vi "create subregions.vi"(8 "error in (no error)":errorcluster, 11 "Autofocus in":refnum<class "Autofocus.lvclass">) -> (0 "error out":errorcluster, 3 "Autofocus out":refnum<class "Autofocus.lvclass">)   [LabVIEW 2012, in "Autofocus.lvclass"]
uses:
  Autofocus.lvclass
  Autofocus.lvclass/Autofocus.ctl
  <vilib>/vision/NI_Vision_Development_Module.lvlib
panel:
  in  "Optional Rectangle":i32[](array[numeric])
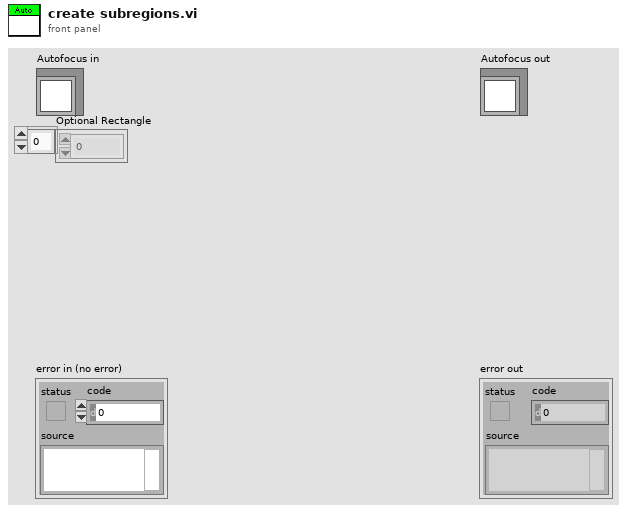
[diagram p1: front panel]
types:
  T1 = typedef "IMAQ Image.ctl" = refnum<image>
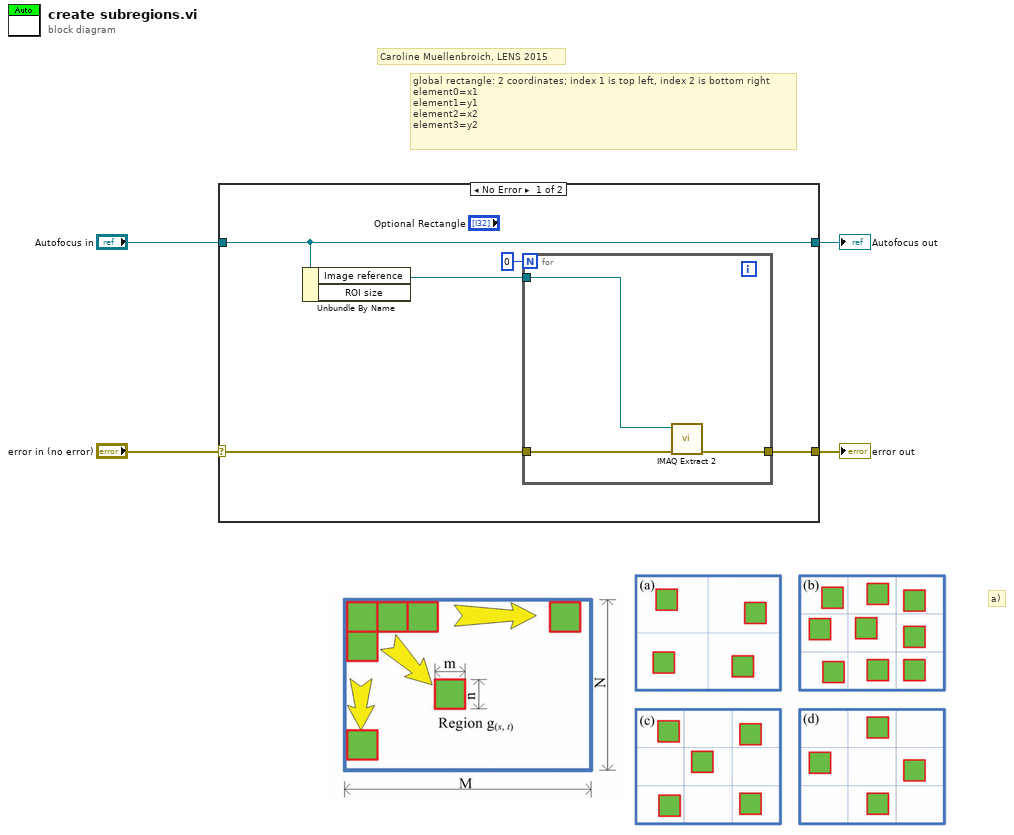
[diagram p0: block diagram]
diagram:
  # "a)"
  # "global rectangle: 2 coordinates; index 1 is top left, index 2 is bottom right\nelement0=x1\nelement1=y1\nelement2=x2\nelement3=y2"
  # "Caroline Muellenbroich, LENS 2015"
  n1 = case shown="No Error" "error in (no error)" {
    selector: "error in (no error)" -> [w7 w14]
    tunnel: [w6 w14] -> w3
    tunnel: [w9 w13] -> w1
    tunnel: "Autofocus in" -> [w9 w13]
    frame No Error {
      n2 = Unbundle By Name(w9) -> ("Image reference"=w8:T1)  [unwired: 1 out]
      n3 = for {
        N: 0 -> [_]
        tunnel: w8 -> [w12]
        tunnel: w7 -> [w11]
        tunnel: [w10] -> w6
        n4 = call "IMAQ Extract 2"("error in (no error)"=w11, "Image Src"=w12) -> ("error out"=w10:errorcluster)  [unwired: 8 in, 1 out]
      }
    }
    frame Error {
    }
  }
  "error out" <- w3
  "Autofocus out" <- w1
